vi "TR_Gen_Empty_Image_with_background.vi"(8 "error in (no error)":errorcluster, 9 "Background color":u32, 10 "Draw Area Size (480 x 480)":T1={"Width"=480, "Height"=480}, 11 "Image Name":string) -> (0 "error out":errorcluster, 3 "Image refnum out":T2)   [LabVIEW 2018, in "Tracks Repair.lvlib"]
uses:
  Tracks Repair.lvlib
  <vilib>/vision/Image Controls.llb/IMAQ Image.ctl
  SubVi's/Controls/CTL_Draw_Area_Size.ctl
  Tracker.lvlib
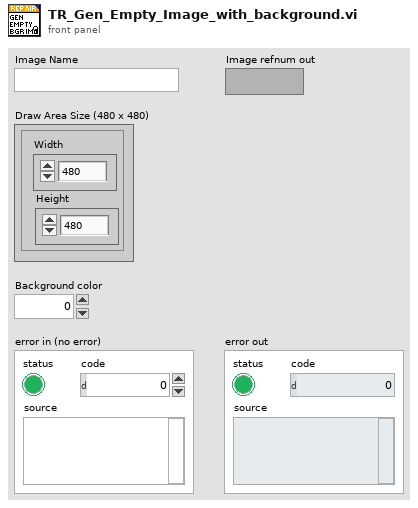
[diagram p1: front panel]
types:
  T1 = typedef "Tracker.lvlib/CTL_Draw_Area_Size.ctl" = cluster{"Width":i32, "Height":i32}
  T2 = typedef "IMAQ Image.ctl" = refnum<image>
  T3 = cluster{"Left":i32, "Top":i32, "Right":i32, "Bottom":i32}
  T4 = typedef "Image Type" = u32
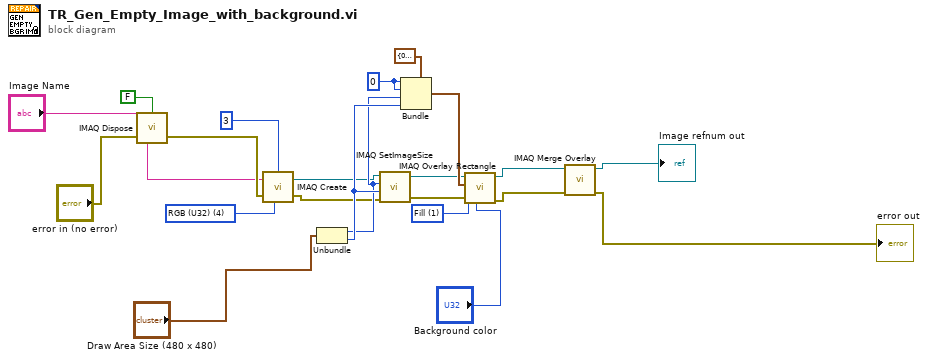
[diagram p0: block diagram]
diagram:
  w14 = 0 ("Left")
  w9 = u32 1 items=["Frame", "Fill", "Highlight"] ("Drawing Mode (Frame)")
  w3 = T4 4 items=["Grayscale (U8)", "Grayscale (I16)", "Grayscale (SGL)", "Complex (CSG)", "RGB (U32)", "HSL (U32)", "RGB (U64)", "Grayscale (U16)"] ("Image Type")
  n1 = call "IMAQ Dispose"("All Images? (No)"=FALSE, "error in (no error)"="error in (no error)") -> ("error out"=w21:errorcluster)  [unwired: 4 in]
  n2 = call "IMAQ Create"("Border Size"=3, "Image Name"="Image Name", "Image Type"=w3, "error in (no error)"=w21) -> ("New Image"=w5:T2, "error out"=w4:errorcluster)  [unwired: 1 in]
  n3 = Unbundle("Draw Area Size (480 x 480)") -> ("Width"=w12:i32, "Height"=w13:i32)
  n4 = call "IMAQ SetImageSize"("error in (no error)"=w4, "Y Resolution"=w13, "X Resolution"=w12, "Image"=w5) -> ("error out"=w6:errorcluster, "Image Out"=w7:T2)  [unwired: 1 in]
  n5 = Bundle(cluster=T3 {"Left"=0, "Top"=0, "Right"=480, "Bottom"=480} ("Rectangle"), "Left"=w14, "Top"=w14, "Right"=w12, "Bottom"=w13) -> (w11:T3)
  n6 = call "IMAQ Overlay Rectangle"("Color"="Background color", "error in (no error)"=w6, "Drawing Mode (Frame)"=w9, "Rectangle"=w11, "Image"=w7) -> ("error out"=w16:errorcluster, "Image Out"=w15:T2)  [unwired: 5 in]
  n7 = call "IMAQ Merge Overlay"("error in (no error)"=w16, "Image Src"=w15) -> ("error out"=→"error out":errorcluster, "Image Dst Out"=→"Image refnum out":T2)  [unwired: 8 in]
